vi "Squareness_1.vi"() -> ()   [LabVIEW 2020]
uses:
  Support/Controls/Clst_Initialize Input.ctl
  Support/Controls/Cmd_Var Data IO.ctl
  Support/Controls/Cmd_Mouse Popup.ctl
  Variables/Global_Cal Info.vi
panel:
  in  "표시방식":string(combo)
  in  "Spec 변경":bool
  in  "Random":bool
  out "Resolution":string[][](table) caption="Spec"
  out "Spec":string[][](table)
  out "제목":string
  out "에러 출력":errorcluster
  out "Condition":string[][](table) caption="2. 직선성 시험"
  in  "최소눈금":string(combo)
  in  "Measured":string[][](table) caption="직각도 측정값 (도)"
  out "Load?":bool
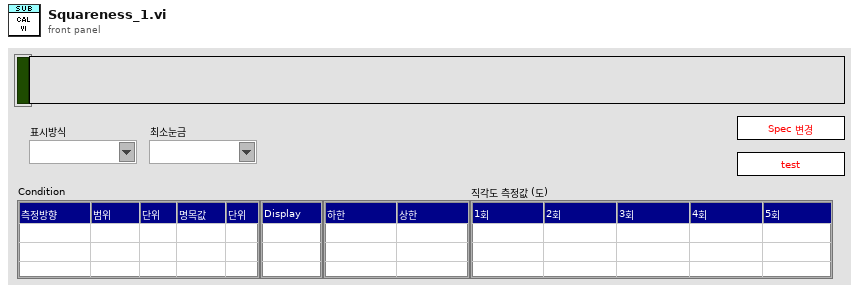
[diagram p1: front panel]
types:
  T1 = typedef "Cmd_Mouse Popup.ctl" = enum16{"활성화", "메뉴선택"}
  T2 = cluster{"Shift":bool, "Ctrl":bool, "Alt":bool, "Cmd":bool, "Opt":bool}
  T3 = typedef "Clst_Initialize Input.ctl" = cluster{"Initialize 1":cluster{"Condition":refnum<vi>[], "Spec":refnum<vi>[], "Measured":refnum<vi>[], "Resolution":refnum<vi>[], "Func_ext":string, "제목":refnum<vi>, "Measured_ADJ":refnum<vi>[]}, "Initialize 2":cluster{"문자열":refnum<vi>[], "콤보박스":refnum<vi>[], "링":refnum<vi>[], "열거형":refnum<vi>[], "테이블":refnum<vi>[], "여러열":refnum<vi>[], "디지털(DBL)":refnum<vi>[], "3D string":refnum<vi>[], "ctrl":refnum<vi>[], "boolean":refnum<vi>[]}}
  T4 = typedef "Cmd_Var Data IO.ctl" = enum16{"Condition", "Condition Default", "Condition_Temp", "Resolution", "Resolution Default", "Resolution Old", "Spec", "Spec Default", "Spec Old", "Spec Temp", "Result", "Result2", "Result3", "Result_Temp", "Result_ADJ", "Result_ADJ2", "STD1", "STD2", "STD3", "STD4", "STD5", "STD Temp", "CMC", "CMC Default"}
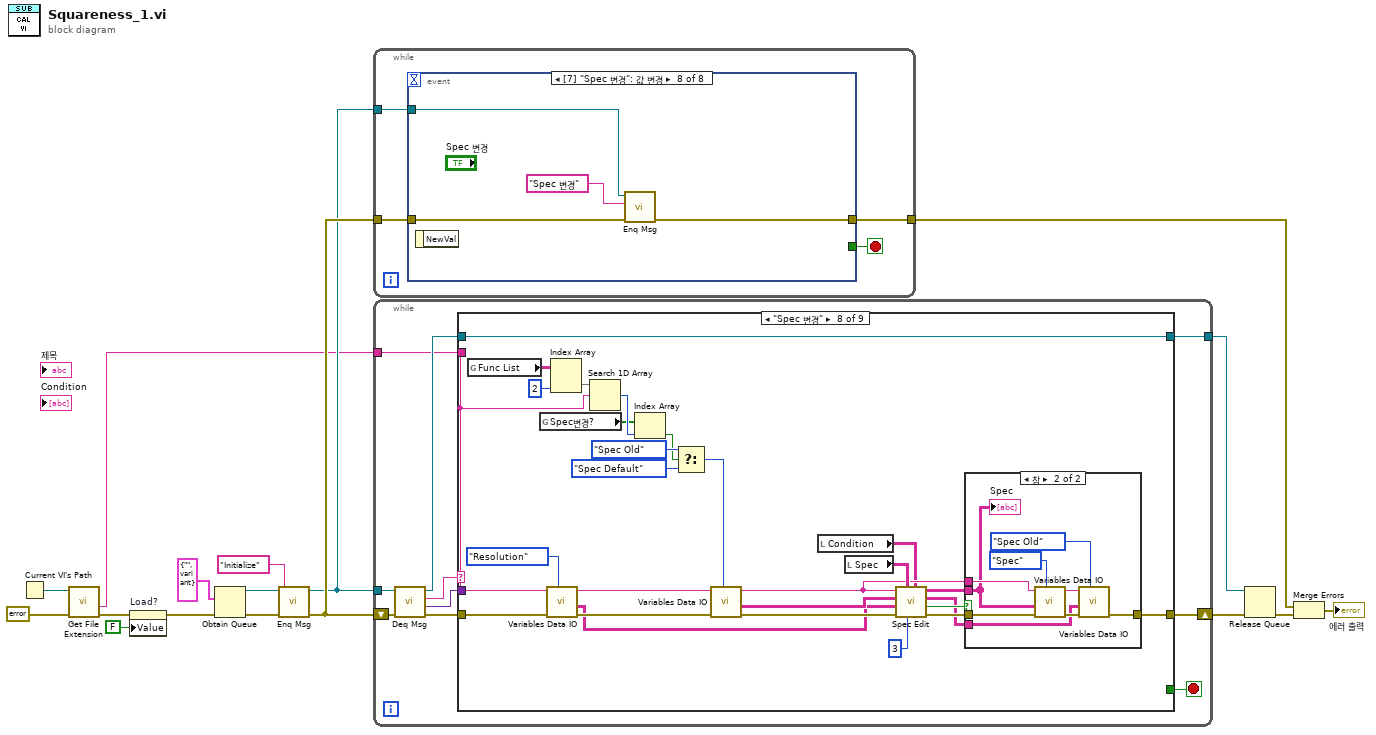
[diagram p0: block diagram]
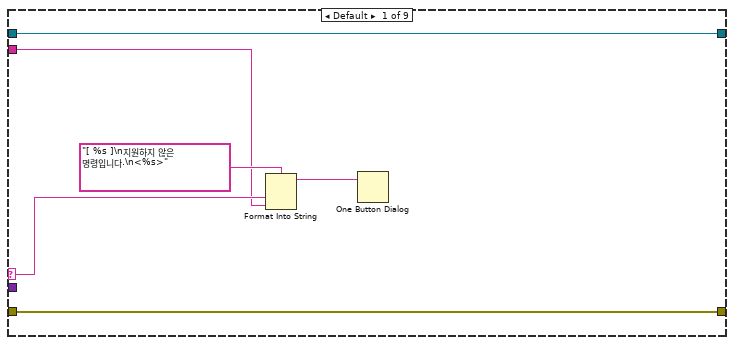
[diagram p2: hidden frame]
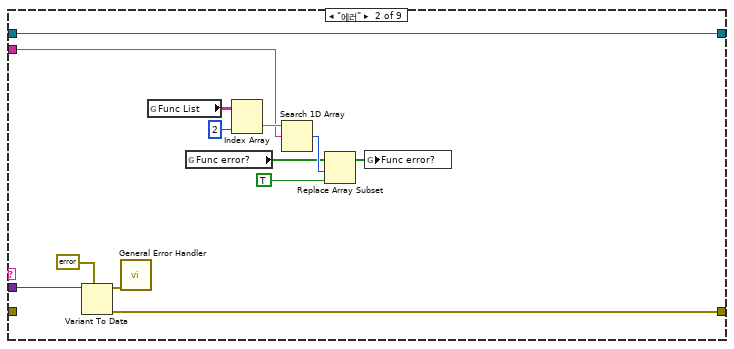
[diagram p3: hidden frame]
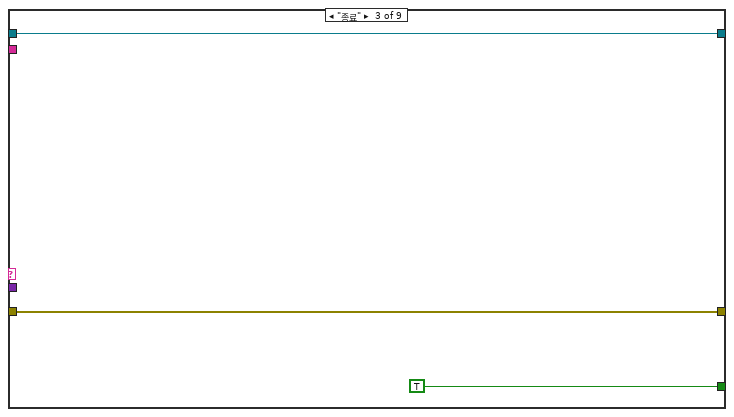
[diagram p4: hidden frame]
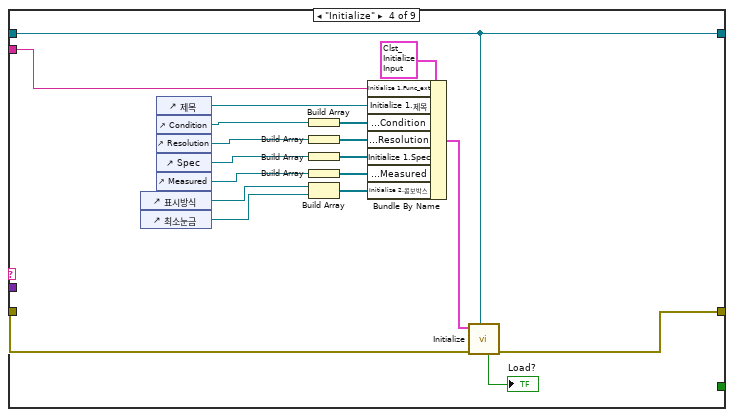
[diagram p5: hidden frame]
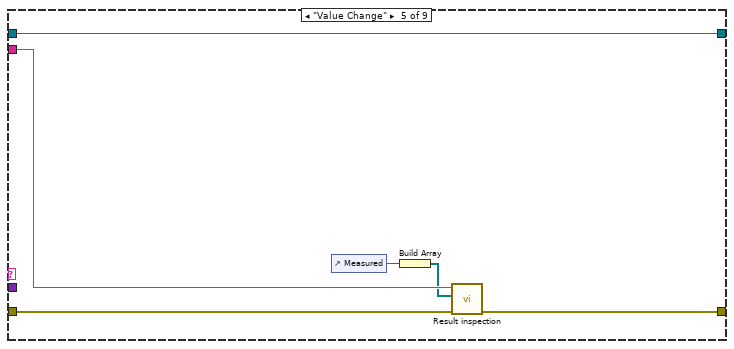
[diagram p6: hidden frame]
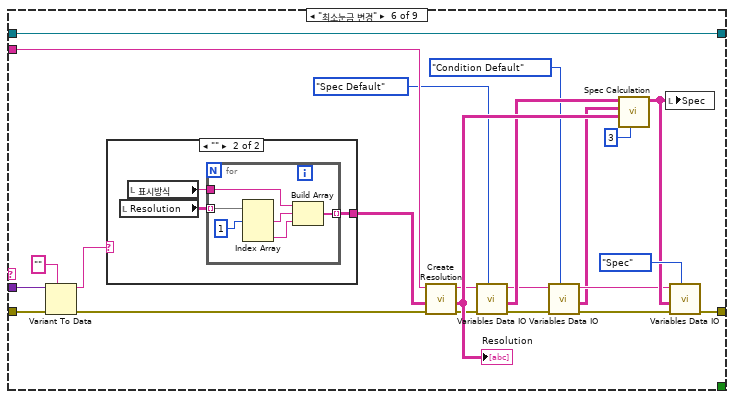
[diagram p7: hidden frame]
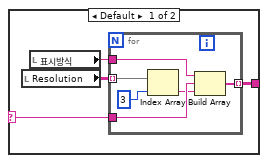
[diagram p8: hidden frame]
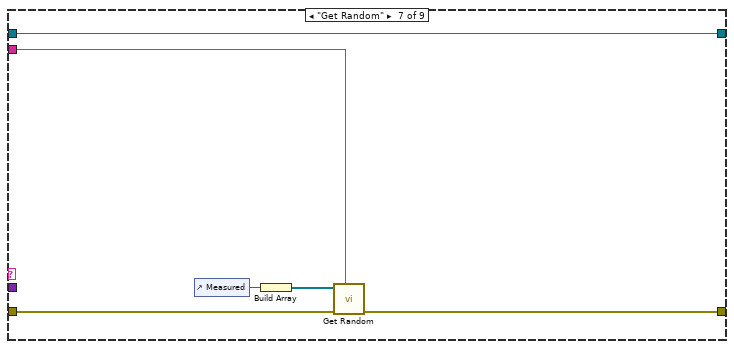
[diagram p9: hidden frame]
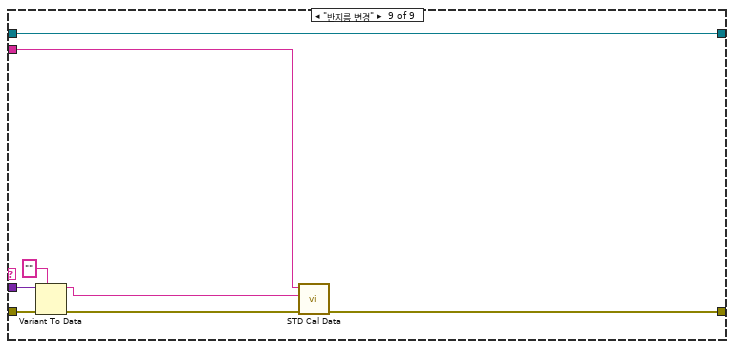
[diagram p11: hidden frame]
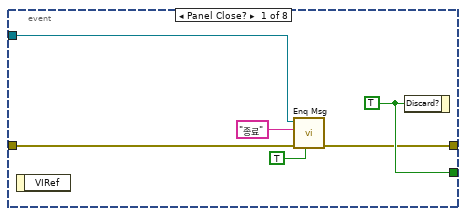
[diagram p12: hidden frame]
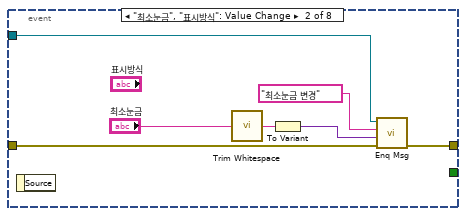
[diagram p13: hidden frame]
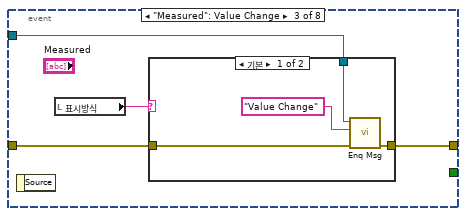
[diagram p14: hidden frame]
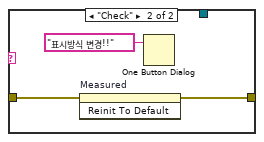
[diagram p15: hidden frame]
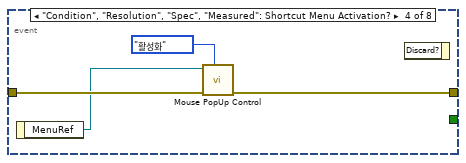
[diagram p16: hidden frame]
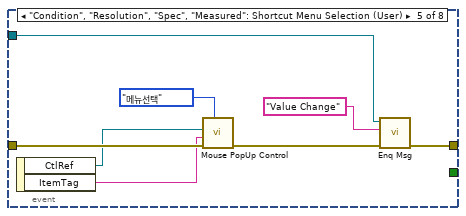
[diagram p17: hidden frame]
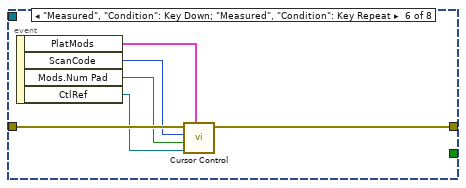
[diagram p18: hidden frame]
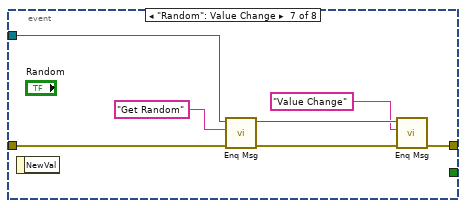
[diagram p19: hidden frame]
diagram:
  n1 = Current VI's Path() -> (path=w5:path)
  n2 = call <vilib>:"Get File Extension.vi"("error in (no error)"=errorcluster {"status"=FALSE, "code"=0, "source"=""} ("에러 상수"), "file"=w5) -> ("error out"=w3:errorcluster, "filename without extension"=w4:string)  [unwired: 5 in, 3 out]
  n3 = property on="Load?" class="Bool (엄격한)"(error in=w3, "Value"=FALSE ("Load?")) -> (error out=w2:errorcluster)  [unwired: 1 in, 1 out]
  n4 = Obtain Queue(element data type=cluster{"메세지":string, "값":variant} {"메세지"="", "값"=variant} ("Message Cluster"), error in (no error)=w2) -> (queue out=w14:refnum<queue>, error out=w16:errorcluster)  [unwired: 3 in, 1 out]
  n5 = call "Enq Msg.vi"("에러 입력(에러 없음)"=w16, "메세지"="Initialize", "큐 입력"=w14) -> ("에러 출력"=w15:errorcluster, "큐 출력"=w12:refnum<queue>)  [unwired: 7 in]
  n6 = while {
    tunnel: w15 -> [w19]
    tunnel: w12 -> [w20]
    tunnel: [w18] -> w9
    stop <- w21 stop-if-true
    n7 = event shown="[7] \"Spec 변경\": 값 변경" {
      selector: _ -> [_ _ _ _ _ _ _ _]
      dyn-events: _ -> [_ _ _ _ _ _ _ _]
      timeout: _ -> [_ _ _ _ _ _ _ _]
      tunnel: [w27 _ _ _ _ _ _ _] -> w21
      tunnel: w20 -> [w25 w33 w38 _ w50 _ w68 w72]
      tunnel: w19 -> [w26 w34 w36 w49 w57 w63 w69 w73]
      tunnel: [w23 w32 w37 w48 w51 w62 w64 w71] -> w18
      event Panel Close? {
        w27 = TRUE ("버림?")
        n8 = event-data() -> ()  [unwired: 1 in, 1 out]
        n9 = call "Enq Msg.vi"("우선순위 메시지?"=TRUE, "에러 입력(에러 없음)"=w26, "메세지"="종료", "큐 입력"=w25) -> ("에러 출력"=w23:errorcluster)  [unwired: 6 in, 1 out]
        n10 = event-data("Discard?"=w27) -> ()  [unwired: 1 in, 1 out]
      }
      event "최소눈금", "표시방식": Value Change {
        n11 = event-data() -> ()  [unwired: 1 in, 1 out]
        n12 = call <vilib>:"Trim Whitespace.vi"("string"="최소눈금") -> ("trimmed string"=w30:string)  [unwired: 1 in]
        n13 = To Variant(anything=w30) -> (Variant=w28:variant)
        n14 = call "Enq Msg.vi"("에러 입력(에러 없음)"=w34, "값"=w28, "메세지"="최소눈금 변경", "큐 입력"=w33) -> ("에러 출력"=w32:errorcluster)  [unwired: 6 in, 1 out]
      }
      event "Measured": Value Change {
        n15 = event-data() -> ()  [unwired: 1 in, 1 out]
        n16 = local read "표시방식"() -> (w35:string)
        n17 = case shown="기본" w35 {
          tunnel: w38 -> [w42 _]
          tunnel: [w41 w43] -> w37
          tunnel: w36 -> [w40 w44]
          frame Default {
            n18 = call "Enq Msg.vi"("에러 입력(에러 없음)"=w40, "메세지"="Value Change", "큐 입력"=w42) -> ("에러 출력"=w41:errorcluster)  [unwired: 7 in, 1 out]
          }
          frame "Check" {
            n19 = invoke on="Measured" class="Tbl (엄격한)" method="Reinit To Default"(error in=w44) -> (error out=w43:errorcluster)  [unwired: 2 in, 2 out]
            n20 = One Button Dialog(message="표시방식 변경!!" ("메시지")) -> ()  [unwired: 1 in, 1 out]
          }
        }
      }
      event "Condition", "Resolution", "Spec", "Measured": Shortcut Menu Activation? {
        n21 = event-data() -> ("MenuRef"=w47:refnum<k9>)  [unwired: 1 in]
        n22 = call "Mouse PopUp Control.vi"("type"=Cmd_Mouse_Popup."활성화", "error in"=w49, "메뉴 참조"=w47) -> ("error out"=w48:errorcluster)  [unwired: 8 in]
        n23 = event-data() -> ()  [unwired: 2 in, 1 out]
      }
      event "Condition", "Resolution", "Spec", "Measured": Shortcut Menu Selection (User) {
        n24 = event-data() -> ("CtlRef"=w55:refnum<vi>, "ItemTag"=w54:string)  [unwired: 1 in]
        n25 = call "Mouse PopUp Control.vi"("type"=Cmd_Mouse_Popup."메뉴선택", "error in"=w57, "아이템 태그"=w54, "Tbl 참조 번호"=w55) -> ("error out"=w52:errorcluster)  [unwired: 7 in]
        n26 = call "Enq Msg.vi"("에러 입력(에러 없음)"=w52, "메세지"="Value Change", "큐 입력"=w50) -> ("에러 출력"=w51:errorcluster)  [unwired: 7 in, 1 out]
      }
      event "Measured", "Condition": Key Down; "Measured", "Condition": Key Repeat {
        n27 = event-data() -> ("PlatMods"=w58:T2, "ScanCode"=w61:i16, "Mods.Num Pad"=w60:bool, "CtlRef"=w59:refnum<vi>)  [unwired: 1 in]
        n28 = call "Cursor Control.vi"("플랫폼 조합키"=w58, "참조"=w59, "Num Pad"=w60, "ScanCode"=w61, "error in"=w63) -> ("error out"=w62:errorcluster)  [unwired: 5 in, 1 out]
      }
      event "Random": Value Change {
        n29 = event-data() -> ()  [unwired: 1 in, 1 out]
        n30 = call "Enq Msg.vi"("에러 입력(에러 없음)"=w69, "메세지"="Get Random", "큐 입력"=w68) -> ("에러 출력"=w67:errorcluster, "큐 출력"=w66:refnum<queue>)  [unwired: 7 in]
        n31 = call "Enq Msg.vi"("에러 입력(에러 없음)"=w67, "메세지"="Value Change", "큐 입력"=w66) -> ("에러 출력"=w64:errorcluster)  [unwired: 7 in, 1 out]
      }
      event "Spec 변경": Value Change {
        n32 = event-data() -> ()  [unwired: 1 in, 1 out]
        n33 = call "Enq Msg.vi"("에러 입력(에러 없음)"=w73, "메세지"="Spec 변경", "큐 입력"=w72) -> ("에러 출력"=w71:errorcluster)  [unwired: 7 in, 1 out]
      }
    }
  }
  n34 = while {
    shift-right: [w84] -> w11
    shift-left: w15 -> [w83]
    tunnel: w12 -> [w81]
    tunnel: [w76] -> w10
    tunnel: w4 -> [w75]
    stop <- w77 stop-if-true
    n35 = call "Deq Msg.vi"("에러 입력(에러 없음)"=w83, "큐 입력"=w81) -> ("에러 출력"=w82:errorcluster, "값"=w78:variant, "메세지"=w80:string, "큐 출력"=w79:refnum<queue>)  [unwired: 6 in]
    n36 = case shown="\"Spec 변경\"" w80 {
      selector: w80 -> [w86 _ _ _ _ _ _ _ _]
      tunnel: w82 -> [w90 _ w106 w125 w128 w153 w175 w199 w223]
      tunnel: [w90 w100 w106 w108 w130 w146 w176 w202 w217] -> w84
      tunnel: w79 -> [w89 w99 w104 w110 w131 w154 w179 w206 w224]
      tunnel: w78 -> [_ w101 _ _ _ w152 _ _ w221]
      tunnel: [_ _ TRUE ("버림?") _ _ _ _ _ _] -> w77
      tunnel: [w89 w99 w104 w110 w131 w154 w179 w206 w224] -> w76
      tunnel: w75 -> [w85 w91 _ w111 w129 w150 w174 w185 w218]
      frame Default {
        n37 = Format Into String(format string="[ %s ]\n지원하지 않은 명령입니다.\n<%s>" ("메시지"), w86, w85) -> (resulting string=w87:string)  [unwired: 2 in, 1 out]
        n38 = One Button Dialog(message=w87) -> ()  [unwired: 1 in, 1 out]
      }
      frame "에러" {
        n39 = Variant To Data(type=errorcluster {"status"=FALSE, "code"=0, "source"=""} ("에러 출력"), Variant=w101) -> (data=w103:errorcluster, error out=w100:errorcluster)  [unwired: 1 in]
        n40 = call <vilib>:"General Error Handler.vi"("error in (no error)"=w103) -> ()  [unwired: 10 in, 5 out]
        n41 = global read "Global_Cal Info.vi" "Func List"() -> (w93:string[][])
        n42 = global read "Global_Cal Info.vi" "Func error?"() -> (w96:bool[])
        n43 = Index Array(array=w93, index (col)=2 ("비활성화된 인덱스 (열)")) -> (element=w94:string[])  [unwired: 1 in]
        n44 = Search 1D Array(1D array=w94, element=w91) -> (index of element=w97:i32)  [unwired: 1 in]
        n45 = Replace Array Subset(array=w96, new element=TRUE ("새 원소/부분배열"), index=w97) -> (w98:bool[])
        n46 = global write "Global_Cal Info.vi" "Func error?"(w98) -> ()
      }
      frame "종료" {
      }
      frame "Initialize" {
        n47 = control-ref of="표시방식"() -> (w109:refnum<vi>)
        n48 = control-ref of="최소눈금"() -> (w118:refnum<vi>)
        n49 = control-ref of="제목"() -> (w116:refnum<vi>)
        n50 = control-ref of="Condition"() -> (w122:refnum<vi>)
        n51 = control-ref of="Resolution"() -> (w112:refnum<vi>)
        n52 = control-ref of="Spec"() -> (w115:refnum<vi>)
        n53 = control-ref of="Measured"() -> (w119:refnum<vi>)
        n54 = Build Array(w122) -> (w121:refnum<vi>[])
        n55 = Build Array(w112) -> (w113:refnum<vi>[])
        n56 = Build Array(w115) -> (w114:refnum<vi>[])
        n57 = Build Array(w119) -> (w120:refnum<vi>[])
        n58 = Build Array(w109, w118) -> (w117:refnum<vi>[])
        n59 = Bundle By Name(cluster=T3 {"Initialize 1"={"Condition"=[], "Spec"=[], "Measured"=[], "Resolution"=[], "Func_ext"="", "제목"=refnum, "Measured_ADJ"=[]}, "Initialize 2"={"문자열"=[], "콤보박스"=[], "링"=[], "열거형"=[], "테이블"=[], "여러열"=[], "디지털(DBL)"=[], "3D string"=[], "ctrl"=[], "boolean"=[]}} ("입력 클러스터"), "Initialize 1.Func_ext"=w111, "Initialize 1.제목"=w116, "Initialize 1.Condition"=w121, "Initialize 1.Resolution"=w113, "Initialize 1.Spec"=w114, "Initialize 1.Measured"=w120, "Initialize 2.콤보박스"=w117) -> (w123:T3)
        n60 = call "Initialize.vi"("큐 입력"=w110, "error in"=w125, "입력 클러스터"=w123) -> ("error out"=w108:errorcluster, "Load?"=→"Load?":bool)  [unwired: 5 in, 2 out]
      }
      frame "Value Change" {
        n61 = control-ref of="Measured"() -> (w127:refnum<vi>)
        n62 = Build Array(w127) -> (w126:refnum<vi>[])
        n63 = call "Result inspection.vi"("error in"=w128, "Ref. Data (Inspection)"=w126, "Func ext"=w129) -> ("error out"=w130:errorcluster)  [unwired: 5 in, 3 out]
      }
      frame "최소눈금 변경" {
        n64 = Variant To Data(error in=w153, type="", Variant=w152) -> (data=w139:string, error out=w141:errorcluster)
        n65 = case shown="\"\"" w139 {
          selector: w139 -> [w155 _]
          tunnel: [w158 w167] -> w140
          frame Default {
            n66 = local read "Resolution"() -> (w157:string[][])
            n67 = local read "표시방식"() -> (w156:string)
            n68 = for {
              tunnel: w157 -> [w164] mode=indexing
              tunnel: w155 -> [w163]
              tunnel: [w161] -> w158 mode=indexing
              tunnel: w156 -> [w160]
              n69 = Index Array(array=w164, index=3 ("인덱스")) -> (element=w162:string)
              n70 = Build Array(w160, w163, w162) -> (w161:string[])
            }
          }
          frame "" {
            n71 = local read "Resolution"() -> (w166:string[][])
            n72 = local read "표시방식"() -> (w165:string)
            n73 = for {
              tunnel: w166 -> [w173] mode=indexing
              tunnel: [w172] -> w167 mode=indexing
              tunnel: w165 -> [w171]
              n74 = Index Array(array=w173, index #1=1 ("인덱스")) -> (element #1=w169:string, element #3=w168:string)  [unwired: 2 in, 1 out]
              n75 = Build Array(w171, w169, w168) -> (w172:string[])
            }
          }
        }
        n76 = call "Create Resolution.vi"("에러 입력(에러 없음)"=w141, "Resolution"=w140, "Func_ext"=w150) -> ("에러 출력"=w144:errorcluster, "Resolution Out"=w147:string[][], "Func_ext 출력"=w143:string)  [unwired: 6 in]
        "Resolution" <- w147
        n77 = call "Variables Data IO.vi"("Select"=Cmd_Var_Data_IO."Spec Default", "error in"=w144, "Func_ext"=w143) -> ("error out"=w135:errorcluster, "Data Out"=w142:string[][], "Func_ext Out"=w136:string)  [unwired: 6 in]
        n78 = call "Variables Data IO.vi"("Select"=Cmd_Var_Data_IO."Condition Default", "error in"=w135, "Func_ext"=w136) -> ("error out"=w133:errorcluster, "Data Out"=w132:string[][], "Func_ext Out"=w134:string)  [unwired: 6 in]
        n79 = call "Spec Calculation.vi"("기준값 열번호"=3 ("열번호(기준값)"), "Resolution"=w147, "Condition in"=w132, "Spec Default"=w142) -> ("Spec out"=w138:string[][])  [unwired: 6 in, 1 out]
        n80 = local write "Spec"(w138) -> ()
        n81 = call "Variables Data IO.vi"("Select"=Cmd_Var_Data_IO."Spec", "error in"=w133, "Data In"=w138, "Func_ext"=w134) -> ("error out"=w146:errorcluster)  [unwired: 5 in, 2 out]
      }
      frame "Get Random" {
        n82 = control-ref of="Measured"() -> (w178:refnum<vi>)
        n83 = Build Array(w178) -> (w177:refnum<vi>[])
        n84 = call "Get Random.vi"("Func_Ext"=w174, "에러 입력"=w175, "Meas"=w177) -> ("에러 출력"=w176:errorcluster)  [unwired: 7 in, 1 out]
      }
      frame "Spec 변경" {
        n85 = global read "Global_Cal Info.vi" "Func List"() -> (w190:string[][])
        n86 = global read "Global_Cal Info.vi" "Spec변경?"() -> (w186:bool[])
        n87 = call "Variables Data IO.vi"("Select"=Cmd_Var_Data_IO."Resolution", "error in"=w199, "Func_ext"=w185) -> ("error out"=w183:errorcluster, "Data Out"=w181:string[][], "Func_ext Out"=w182:string)  [unwired: 6 in]
        n88 = Index Array(array=w190, index (col)=2 ("비활성화된 인덱스 (열)")) -> (element=w188:string[])  [unwired: 1 in]
        n89 = Search 1D Array(1D array=w188, element=w185) -> (index of element=w187:i32)  [unwired: 1 in]
        n90 = Index Array(array=w186, index=w187) -> (element=w191:bool)
        n91 = Select(t=Cmd_Var_Data_IO."Spec Old" ("Select"), s=w191, f=Cmd_Var_Data_IO."Spec Default" ("Select")) -> (s? t:f=w184:T4)
        n92 = call "Variables Data IO.vi"("Select"=w184, "error in"=w183, "Func_ext"=w182) -> ("error out"=w201:errorcluster, "Data Out"=w194:string[][], "Func_ext Out"=w195:string)  [unwired: 6 in]
        n93 = local read "Condition"() -> (w180:string[][])
        n94 = local read "Spec"() -> (w196:string[][])
        n95 = call "Spec Edit.vi"("Condition"=w180, "열번호(기준값)"=3, "Spec Value"=w196, "에러 입력(에러 없음)"=w201, "Resolution"=w181, "Spec Default"=w194, "Func_ext"=w195) -> ("에러 출력"=w203:errorcluster, "변경?"=w204:bool, "Spec Default out"=w198:string[][], "Spec 출력"=w205:string[][])  [unwired: 1 in]
        n96 = case shown="참" w204 {
          tunnel: w205 -> [_ w213]
          tunnel: w203 -> [w207 w216]
          tunnel: [w207 w211] -> w202
          tunnel: w195 -> [_ w214]
          tunnel: w198 -> [_ w209]
          frame False {
          }
          frame True {
            n97 = call "Variables Data IO.vi"("Select"=Cmd_Var_Data_IO."Spec", "error in"=w216, "Data In"=w213, "Func_ext"=w214) -> ("error out"=w212:errorcluster, "Func_ext Out"=w210:string)  [unwired: 5 in, 1 out]
            n98 = call "Variables Data IO.vi"("Select"=Cmd_Var_Data_IO."Spec Old", "error in"=w212, "Data In"=w209, "Func_ext"=w210) -> ("error out"=w211:errorcluster)  [unwired: 5 in, 2 out]
            "Spec" <- w213
          }
        }
      }
      frame "반지름 변경" {
        n99 = Variant To Data(error in=w223, type="", Variant=w221) -> (data=w219:string, error out=w222:errorcluster)
        n100 = call "STD Cal Data.vi"("error in"=w222, "문자열"=w219, "Func_ext"=w218) -> ("error out"=w217:errorcluster)  [unwired: 4 in, 4 out]
      }
    }
  }
  n101 = Release Queue(queue=w10, error in (no error)=w11) -> (error out=w8:errorcluster)  [unwired: 1 in, 2 out]
  n102 = Merge Errors(w9, w8) -> (→"에러 출력":errorcluster)
